vi "ChangeMusicVolume.vi"(8 "error in (no error)":errorcluster, 10 "VolumeData":T1, 11 "Game in":refnum<class "Game.lvclass">) -> (0 "error out":errorcluster, 3 "Game out":refnum<class "Game.lvclass">)   [LabVIEW 2019, in "RT_Game.lvlib" / "Game.lvclass"]
uses:
  Game.lvclass
  Engine/ChangeVolumeData.ctl
  Engine/MessageCluster.ctl
  Game.lvclass/Game.ctl
  Engine/Engine.lvclass
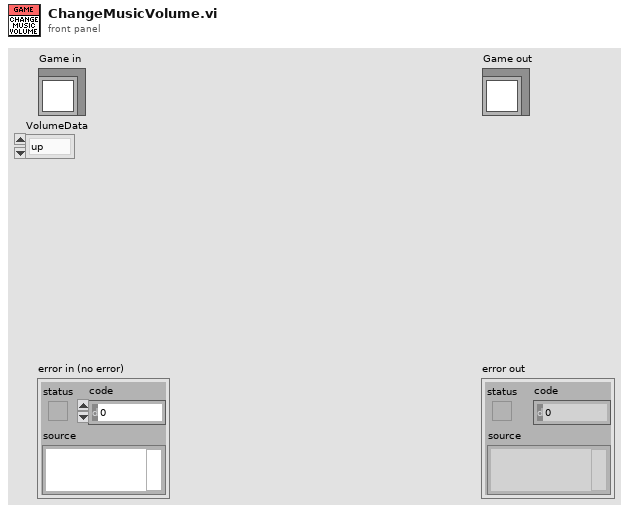
[diagram p1: front panel]
types:
  T1 = typedef "RT_Game.lvlib/Engine.lvclass/ChangeVolumeData.ctl" = enum16{"up", "down", "mute"}
  T2 = typedef "RT_Game.lvlib/Engine.lvclass/MessageCluster.ctl" = cluster{"Message":string, "Data":variant}
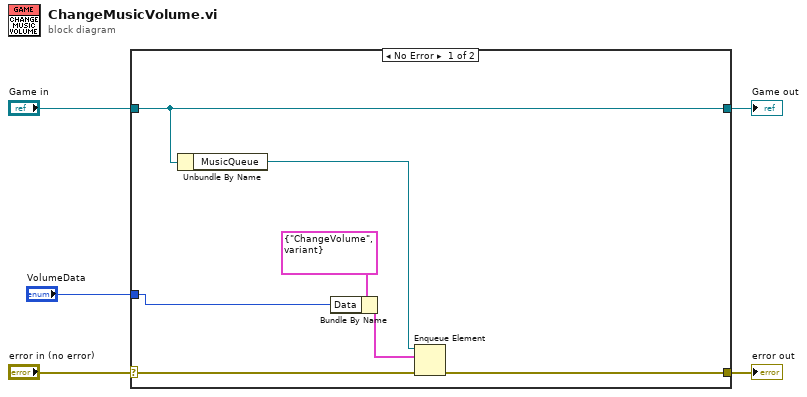
[diagram p0: block diagram]
diagram:
  n1 = case shown="No Error" "error in (no error)" {
    selector: "error in (no error)" -> [w12 w14]
    tunnel: [w10 w14] -> w4
    tunnel: [w11 w13] -> w2
    tunnel: "Game in" -> [w11 w13]
    tunnel: "VolumeData" -> [w6 _]
    frame No Error {
      n2 = Unbundle By Name(w11) -> ("MusicQueue"=w9:refnum<queue>)
      n3 = Bundle By Name(cluster=T2 {"Message"="ChangeVolume", "Data"=variant} ("element"), "Data"=w6) -> (w7:T2)
      n4 = Enqueue Element(queue=w9, element=w7, error in (no error)=w12) -> (error out=w10:errorcluster)  [unwired: 1 in, 2 out]
    }
    frame Error {
    }
  }
  "error out" <- w4
  "Game out" <- w2
